vi "BoxMuller.vi"(8 "error in (no error)":errorcluster, 11 "RSA in":refnum<class "RSA.lvclass">) -> (0 "error out":errorcluster, 1 "random2":dbl, 2 "random1":dbl, 3 "RSA out":refnum<class "RSA.lvclass">)   [LabVIEW 2012, in "RSA.lvclass"]
uses:
  RSA.lvclass
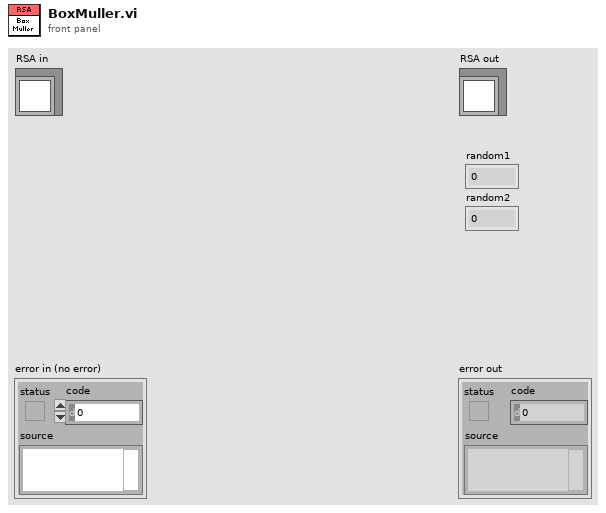
[diagram p1: front panel]
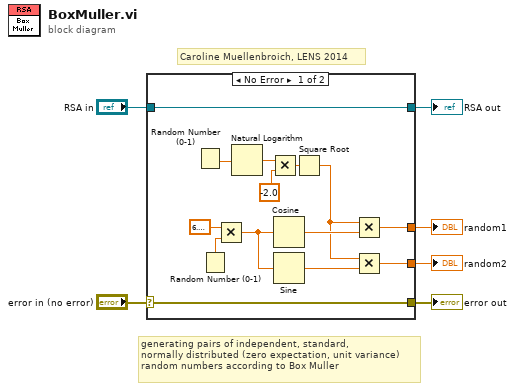
[diagram p0: block diagram]
diagram:
  # "Caroline Muellenbroich, LENS 2014"
  # "generating pairs of independent, standard,\nnormally distributed (zero expectation, unit variance)\nrandom numbers according to Box Muller"
  n1 = case shown="No Error" "error in (no error)" {
    selector: "error in (no error)" -> [w19 w22]
    tunnel: [w19 w22] -> w5
    tunnel: [w20 w21] -> w3
    tunnel: "RSA in" -> [w20 w21]
    tunnel: [w8 _] -> w2
    tunnel: [w7 _] -> w1
    frame No Error {
      n2 = Random Number (0-1)() -> (number: 0 to 1=w16:dbl)
      n3 = Random Number (0-1)() -> (number: 0 to 1=w14:dbl)
      n4 = Multiply(x=6.283185307179586, y=w14) -> (x*y=w11:dbl)
      n5 = Natural Logarithm(1:w16) -> (0:w17:dbl)
      n6 = Multiply(x=w17, y=-2.0 ("x")) -> (x*y=w15:dbl)
      n7 = Cosine(x=w11) -> (cos(x)=w12:dbl)
      n8 = Sine(x=w11) -> (sin(x)=w10:dbl)
      n9 = Square Root(x=w15) -> (sqrt(x)=w9:dbl)
      n10 = Multiply(x=w9, y=w12) -> (x*y=w8:dbl)
      n11 = Multiply(x=w9, y=w10) -> (x*y=w7:dbl)
    }
    frame Error {
    }
  }
  "error out" <- w5
  "RSA out" <- w3
  "random1" <- w2
  "random2" <- w1
